vi "SF2_BUFFER.vi"(5 "Device Number":T1, 9 "Buffer Time (sec)":dbl=10.0 format="%#_13g", 11 "Sample rate":u8=50) -> ()   [LabVIEW 2016]
uses:
  <userlib>/labviewae/_TypeDefs/FRIC_navX_DeviceNumbersTypeDef.ctl
  _Process_Loop/FRIC_SF2_Process Loop TypeDef.ctl
  _Process_Loop/FRIC_SF2_ProcessingLoopStatesTypeDef_I2C.ctl
  _Notifier/SF2_NotifyPacketTypeDef.ctl
  _Notifier/SF2_ActionTypeDef.ctl
  <vilib>/Platform/TimedLoop/XDataNode/timing_clust.ctl
  <vilib>/Platform/TimedLoop/XDataNode/nitl_modes.ctl
  <vilib>/Platform/TimedLoop/XDataNode/wakeup.ctl
  <vilib>/Platform/TimedLoop/XDataNode/XDataNode.xnode
  <vilib>/Platform/TimedLoop/XDataNode/XDNodeRunTimeDep.lvlib
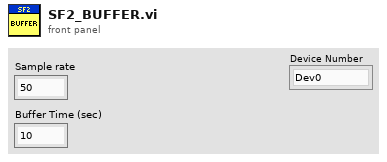
[diagram p1: front panel]
types:
  T1 = typedef "FRIC_navX_DeviceNumbersTypeDef.ctl" = enum16{"Dev0", "Dev1", "Dev2", "Dev3", "Dev4", "Dev5", "Dev6", "Dev7", "Dev8", "Dev9", "Dev10"}
  T2 = typedef "FRIC_SF2_Process Loop TypeDef.ctl" = cluster{"State Array":T3[], "error":errorcluster, "SF2 Buffer":dbl[][], "Loop Frequency":u32, "Buffer Size":dbl, "notifier ref out":refnum<notifier>, "Sample rate":u8}
  T3 = typedef "FRIC_SF2_ProcessingLoopStatesTypeDef_I2C.ctl" = enum16{"Process", "Hault", "Exit", "VI_INI"}
  T4 = typedef "XDNodeRunTimeDep.lvlib/timing_clust.ctl" = cluster{"Expected End [f-1]":u64, "Actual End [f-1]":u64, "Finished Late? [f-1]":bool, "Expected End [i-1]":u64, "Actual End [i-1]":u64, "Finished Late? [i-1]":bool, "Expected Start [i]":u64, "Actual Start [i]":u64, "Expected Start [f]":u64, "Actual Start [f]":u64, "Source Name":string, "Structure Name":string, "Period":i64, "Deadline":i64, "Offset":i64, "Start":i64, "Priority":i32, "Timeout":i32, "Mode":T5, "Wakeup Reason":T6, "Error":errorcluster, "Source Type":string, "Secondary Source Type":string, "Global End Time":u64, "Global Start Time":u64, "Frame Duration":u64, "Iteration Duration":u64, "Assigned CPU":i32, "I/O Scan Engine Mode":u32}
  T5 = typedef "XDNodeRunTimeDep.lvlib/nitl_modes.ctl" = enum32{"No Change", "Process missed periods, maintain original phase", "Discard missed periods, maintain original phase", "Process missed periods, ignore original phase", "Discard missed periods, ignore original phase"}
  T6 = typedef "XDNodeRunTimeDep.lvlib/wakeup.ctl" = enum32{"Normal", "Aborted", "Asynchronous wakeup", "Timing source error", "Timed loop error", "Timeout"}
  T7 = typedef "SF2_NotifyPacketTypeDef.ctl" = cluster{"SF2 Action":T8, "Data":variant}
  T8 = typedef "SF2_ActionTypeDef.ctl" = enum16{"None", "Halt", "Reset Buffer"}
  T9 = cluster{"Quat W":dbl, "Quat X":dbl, "Quat Y":dbl, "Quat Z":dbl}
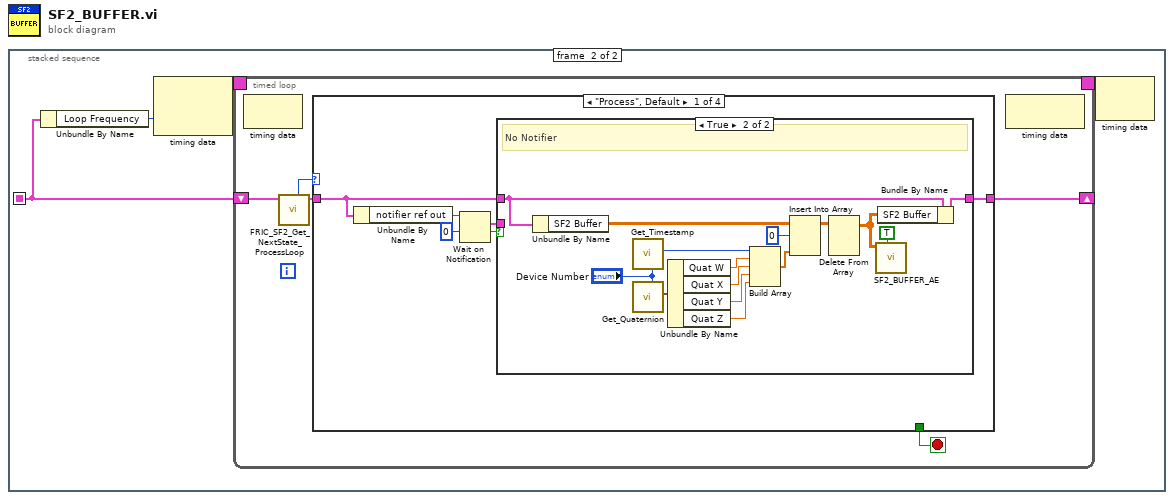
[diagram p0: block diagram]
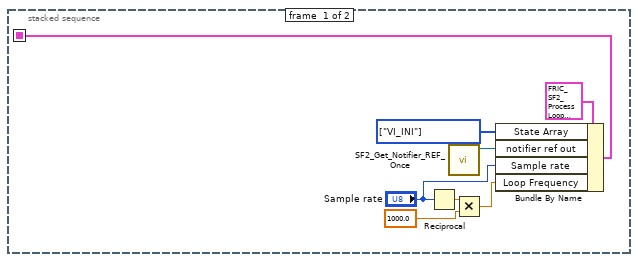
[diagram p2: hidden frame]
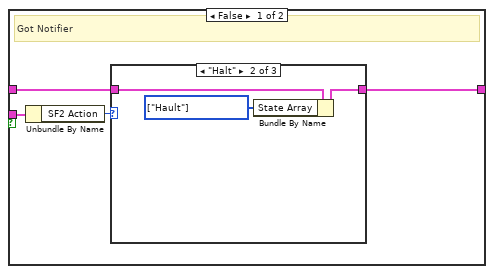
[diagram p3: hidden frame]
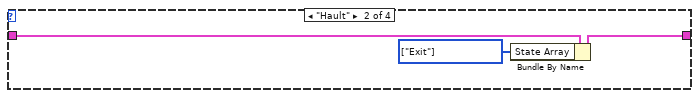
[diagram p6: hidden frame]
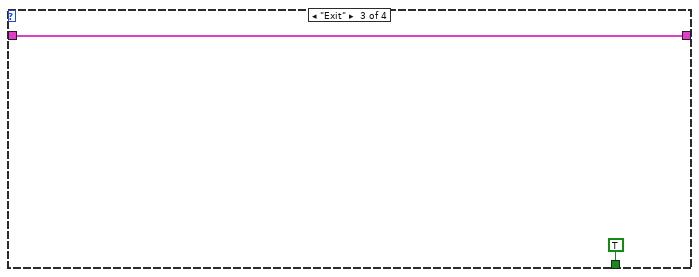
[diagram p7: hidden frame]
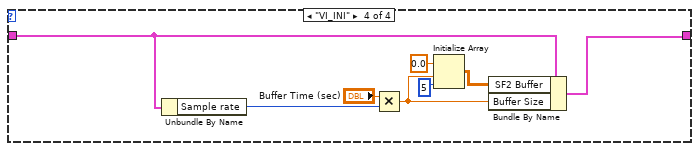
[diagram p8: hidden frame]
diagram:
  n1 = stacked-sequence {
    seq-local: [w7 _] -> [_ w10]
    frame #0 {
      w5 = T3[] [enum."VI_INI"] items=["Process", "Hault", "Exit", "VI_INI"] ("State Array")
      n2 = Reciprocal(x="Sample rate") -> (1/x=w4:dbl)
      n3 = call "SF2_Get_Notifier_REF_Once.vi"() -> ("notifier ref out"=w6:refnum<notifier>)  [unwired: 10 in, 1 out]
      n4 = Multiply(x=w4, y=1000.0) -> (x*y=w2:dbl)
      n5 = Bundle By Name(cluster=T2 {"State Array"=[enum."Hault", enum."Process"], "error"={"status"=FALSE, "code"=0, "source"=""}, "SF2 Buffer"=[], "Loop Frequency"=200, "Buffer Size"=2000.0, "notifier ref out"=refnum, "Sample rate"=200} ("SF2 Process Loop TypeDef (out)"), "State Array"=w5, "notifier ref out"=w6, "Sample rate"="Sample rate", "Loop Frequency"=w2) -> (w7:T2)
    }
    frame #1 {
      n6 = Unbundle By Name(w10) -> ("Loop Frequency"=w9:u32)
      n7 = node-c288(w9) -> (w12:T4)  [unwired: 1 in]
      n8 = timed-loop {
        shift-right: [w14] -> _
        shift-left: w10 -> [w16]
        timing: w12 -> [_]
        timing-out: [_] -> w11
        stop <- w17 stop-if-true
        n9 = node-c288() -> ()  [unwired: 1 in, 1 out]
        n10 = call "FRIC_SF2_Get_NextState_ProcessLoop.vi"("SF2 Process Loop TypeDef (in)"=w16) -> ("SF2 Process Loop TypeDef (out)"=w15:T2, "Current State"=w13:T3)  [unwired: 9 in]
        n11 = case shown="\"Process\", Default" w13 {
          tunnel: [_ _ TRUE _] -> w17
          tunnel: w15 -> [w25 w52 w54 w56]
          tunnel: [w24 w51 w54 w61] -> w14
          frame "Process", Default {
            n12 = Unbundle By Name(w25) -> ("notifier ref out"=w22:refnum<notifier>)
            n13 = Wait on Notification(notifier=w22, timeout in ms (-1)=0) -> (notification=w20:T7, timed out?=w21:bool)  [unwired: 2 in, 2 out]
            n14 = case shown="True" w21 {
              tunnel: [w27 w45] -> w24
              tunnel: w25 -> [w28 w44]
              tunnel: w20 -> [w29 _]
              frame False {
                # "Got Notifier"
                n15 = Unbundle By Name(w29) -> ("SF2 Action"=w26:T8)
                n16 = case shown="\"Halt\"" w26 {
                  tunnel: w28 -> [w30 w33 w34]
                  tunnel: [w30 w32 w34] -> w27
                  frame "None", Default {
                  }
                  frame "Halt" {
                    w31 = T3[] [enum."Hault"] items=["Process", "Hault", "Exit", "VI_INI"] ("State Array")
                    # "Got Notifier"
                    n17 = Bundle By Name(cluster=w33, "State Array"=w31) -> (w32:T2)
                  }
                  frame "Reset Buffer" {
                  }
                }
              }
              frame True {
                # "No Notifier"
                n18 = Unbundle By Name(w44) -> ("SF2 Buffer"=w46:dbl[][])
                n19 = call <userlib>:"Get_Timestamp.vi"("Device Number"="Device Number") -> ("Timestamp"=w43:u32)  [unwired: 10 in]
                n20 = call <userlib>:"Get_Quaternion.vi"("Device Number"="Device Number") -> ("Quaternion"=w47:T9)  [unwired: 10 in]
                n21 = Unbundle By Name(w47) -> ("Quat W"=w42:dbl, "Quat X"=w41:dbl, "Quat Y"=w40:dbl, "Quat Z"=w39:dbl)
                n22 = Build Array(w43, w42, w41, w40, w39) -> (w38:dbl[])
                n23 = Insert Into Array(array=w46, index (row)=0 ("index"), new element=w38) -> (w49:dbl[][])  [unwired: 1 in]
                n24 = Delete From Array(array=w49) -> (array with subset deleted=w37:dbl[][])  [unwired: 3 in, 1 out]
                n25 = call "SF2_BUFFER_AE.vi"("Update"=TRUE, "SF2 Buffer (in)"=w37) -> ()  [unwired: 9 in, 1 out]
                n26 = Bundle By Name(cluster=w44, "SF2 Buffer"=w37) -> (w45:T2)
              }
            }
          }
          frame "Hault" {
            w50 = T3[] [enum."Exit"] items=["Process", "Hault", "Exit", "VI_INI"] ("State Array")
            n27 = Bundle By Name(cluster=w52, "State Array"=w50) -> (w51:T2)
          }
          frame "Exit" {
          }
          frame "VI_INI" {
            n28 = Unbundle By Name(w56) -> ("Sample rate"=w55:u8)
            n29 = Multiply(x="Buffer Time (sec)", y=w55) -> (x*y=w58:dbl)
            n30 = Initialize Array(0.0 ("Numeric"), w58, 5 ("dimension size")) -> (w59:dbl[][])
            n31 = Bundle By Name(cluster=w56, "SF2 Buffer"=w59, "Buffer Size"=w58) -> (w61:T2)
          }
        }
        n32 = node-c288() -> ()  [unwired: 1 in, 1 out]
      }
      n33 = node-c288(w11) -> ()  [unwired: 1 out]
    }
  }
